vi "rs3_2D Plane fit_sub4.vi"(0 "Pointcloud X":dbl[][](array[numeric]), 1 "method":T2 items=["Least Square", "Least Absolute Residual", "Bisquare"], 5 "Pointcloud Y":dbl[][](array[numeric]), 9 "Pointcloud Z":dbl[][](array[numeric]), 12 "algorithm":T1 items=["SVD", "Givens", "Givens2", "Householder", "LU Decomposition", "Cholesky", "SVD for Rank Deficient H"]) -> (2 "AngleX":dbl=1.3187701159862044 format="%0.8f", 3 "Best Fit":dbl[](array[numeric])=[5.060084925690024, 5.062845010615716, 5.065605095541407, 5.0435244161358845, 5.046284501061575, 5.049044585987266, 5.026963906581743, 5.029723991507435, 5.015923566878985], 4 "rms %":dbl=1.3187701159862044 format="%0.4f", 6 "rms error value":dbl=0.06652497327232935 format="%0.4f", 8 "error":i32, 10 "mean Z Value":dbl=5.04447078879859 format="%0.2f", 11 "Raw RMS%":dbl format="%0.2f", 13 "AngleY":dbl=1.3187701159862044 format="%0.8f", 14 "Deviation":dbl[](array[numeric])=[-0.060084925690023994, 0.037154989384283965, 0.03439490445859228, 0.05647558386411511, -0.14628450106157498, 0.05095541401273351, 0.07303609341825634, -0.029723991507434988, -0.01592356687898544], 15 "Coefficients":dbl[](array[numeric])=[5.057324840764333, 0.002760084925691242, -0.016560509554140346])   [LabVIEW 2017, in "libRealSense3.lvlib"]
uses:
  libRealSense3.lvlib
  <vilib>/Analysis/6fits.llb/Curve Fitting Criteria.ctl
  <vilib>/Analysis/6fits.llb/General Linear Fit Algorithm.ctl
  <vilib>/Analysis/baseanly.llb/Mean (DBL).vi
  <vilib>/Analysis/5stat.llb/RMS (DBL).vi
  <vilib>/Analysis/NI_AALPro.lvlib
  <vilib>/Analysis/NI_AALBase.lvlib
panel:
  # "INPUT DATA"
  # "PLANE FIT"
  # "Z= A +B*x+C*y"
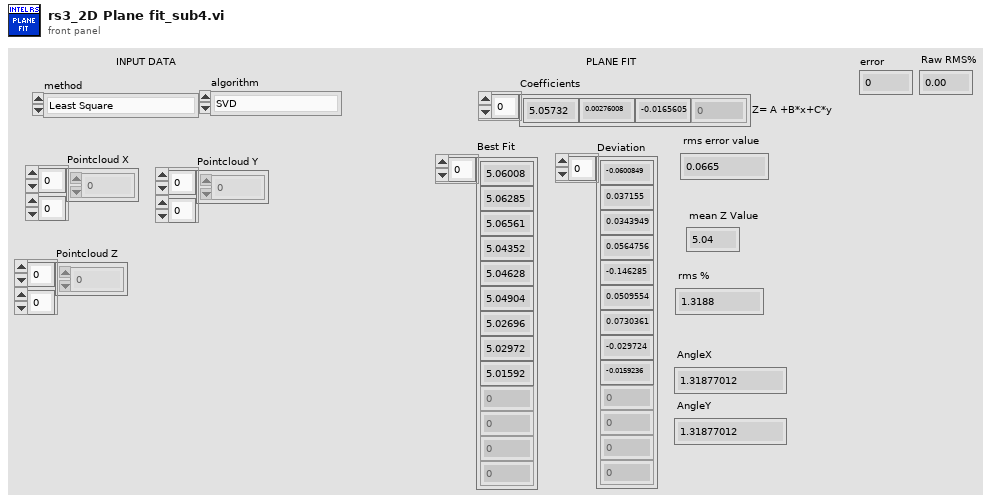
[diagram p1: front panel]
types:
  T1 = typedef "NI_AALPro.lvlib/General Linear Fit Algorithm.ctl" = u16
  T2 = typedef "NI_AALPro.lvlib/Curve Fitting Criteria.ctl" = u16
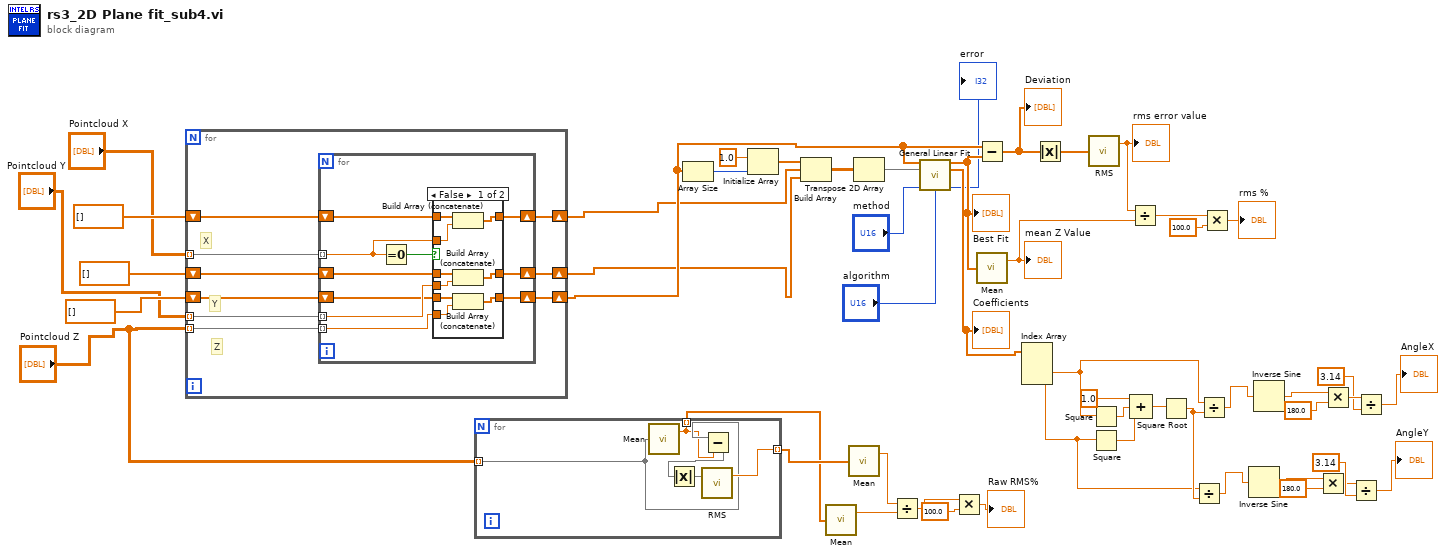
[diagram p0: block diagram]
diagram:
  n1 = for {
    tunnel: "Pointcloud X" -> [w61] mode=indexing
    tunnel: "Pointcloud Y" -> [w60] mode=indexing
    tunnel: "Pointcloud Z" -> [w59] mode=indexing
    shift-right: [w58] -> w30
    shift-left: dbl[] [] -> [w55]
    shift-right: [w56] -> w31
    shift-left: dbl[] [] -> [w54]
    shift-right: [w57] -> w32
    shift-left: dbl[] [] -> [w53]
    # "Z"
    # "Y"
    # "X"
    n2 = for {
      tunnel: w61 -> [w70] mode=indexing
      tunnel: w60 -> [w67] mode=indexing
      tunnel: w59 -> [w66] mode=indexing
      shift-right: [w69] -> w58
      shift-left: w55 -> [w68]
      shift-right: [w63] -> w56
      shift-left: w54 -> [w62]
      shift-right: [w64] -> w57
      shift-left: w53 -> [w65]
      n3 = Equal To 0?(x=w70) -> (x = 0?=w71:bool)
      n4 = case shown="False" w71 {
        tunnel: w70 -> [w80 _]
        tunnel: [w79 w83] -> w69
        tunnel: w68 -> [w78 w83]
        tunnel: w67 -> [w77 _]
        tunnel: w66 -> [w76 _]
        tunnel: w65 -> [w75 w81]
        tunnel: [w74 w81] -> w64
        tunnel: [w73 w82] -> w63
        tunnel: w62 -> [w72 w82]
        frame False {
          n5 = Build Array (concatenate)(w78, w80) -> (w79:dbl[])
          n6 = Build Array (concatenate)(w72, w77) -> (w73:dbl[])
          n7 = Build Array (concatenate)(w75, w76) -> (w74:dbl[])
        }
        frame True {
        }
      }
    }
  }
  n8 = for {
    tunnel: "Pointcloud Z" -> [w85] mode=indexing
    tunnel: [w88] -> w7 mode=indexing
    tunnel: [w84] -> w5 mode=indexing
    n9 = call-poly <vilib>:"Mean.vi"("X"=w85) -> ("mean"=w84:dbl)  [unwired: 1 out]
    n10 = Subtract(x=w85, y=w84) -> (x-y=w87:dbl[])
    n11 = Absolute Value(x=w87) -> (abs(x)=w86:dbl[])
    n12 = call-poly <vilib>:"RMS.vi"("X"=w86) -> ("rms value"=w88:dbl)  [unwired: 1 out]
  }
  n13 = Array Size(array=w32) -> (size(s)=w52:i32)
  n14 = Initialize Array(1.0 ("element"), w52) -> (w50:dbl[])
  n15 = Build Array(w50, w30, w31) -> (w38:dbl[][])
  n16 = call-poly <vilib>:"Mean.vi"("X"=w5) -> ("mean"=w4:dbl)  [unwired: 1 out]
  n17 = call-poly <vilib>:"Mean.vi"("X"=w7) -> ("mean"=w6:dbl)  [unwired: 1 out]
  n18 = Transpose 2D Array(2D array=w38) -> (transposed array=w49:dbl[][])
  n19 = Divide(x=w6, y=w4) -> (x/y=w2:dbl)
  n20 = call <vilib>:"General Linear Fit.vi"("Y"=w32, "H"=w49, "method"="method", "algorithm"="algorithm") -> ("Best Fit"=w44:dbl[], "Coefficients"=w29:dbl[], "error"=→"error":i32)  [unwired: 6 in, 3 out]
  "Best Fit" <- w44
  "Coefficients" <- w29
  n21 = Multiply(x=w2, y=100.0) -> (x*y=→"Raw RMS%":dbl)
  n22 = Subtract(x=w32, y=w44) -> (x-y=w46:dbl[])
  "Deviation" <- w46
  n23 = call-poly <vilib>:"Mean.vi"("X"=w44) -> ("mean"=w42:dbl)  [unwired: 1 out]
  "mean Z Value" <- w42
  n24 = Index Array(array=w29) -> (element #2=w10:dbl, element #3=w11:dbl)  [unwired: 3 in, 1 out]
  n25 = Absolute Value(x=w46) -> (abs(x)=w45:dbl[])
  n26 = call-poly <vilib>:"RMS.vi"("X"=w45) -> ("rms value"=w43:dbl)  [unwired: 1 out]
  "rms error value" <- w43
  n27 = Square(x=w10) -> (x^2=w21:dbl)
  n28 = Square(x=w11) -> (x^2=w27:dbl)
  n29 = Divide(x=w43, y=w42) -> (x/y=w41:dbl)
  n30 = Compound Arithmetic op=ADD(1.0 ("value"), w21, w27) -> (w28:dbl)
  n31 = Square Root(x=w28) -> (sqrt(x)=w14:dbl)
  n32 = Divide(x=w11, y=w14) -> (x/y=w15:dbl)
  n33 = Divide(x=w10, y=w14) -> (x/y=w26:dbl)
  n34 = Multiply(x=w41, y=100.0) -> (x*y=→"rms %":dbl)
  n35 = Inverse Sine(1:w15) -> (0:w16:dbl)
  n36 = Inverse Sine(1:w26) -> (0:w25:dbl)
  n37 = Multiply(x=w16, y=180.0) -> (x*y=w18:dbl)
  n38 = Multiply(x=w25, y=180.0) -> (x*y=w23:dbl)
  n39 = Divide(x=w18, y=3.14) -> (x/y=→"AngleY":dbl)
  n40 = Divide(x=w23, y=3.14) -> (x/y=→"AngleX":dbl)
